vi "start.search.vi"(8 "error in (no error)":errorcluster, 9 "search dirs":path[](array[path]), 11 "comic_crawler in":refnum<class "comic_crawler.lvclass">) -> (0 "error out":errorcluster, 3 "comic_crawler out":refnum<class "comic_crawler.lvclass">)   [LabVIEW 2024, in "comic_crawler.lvclass"]
uses:
  comic_crawler.lvclass
  daemon.states--enum.ctl
  WebScraper/comic_class/comic_class.lvclass
  comic_crawler.lvclass/comic_crawler.ctl
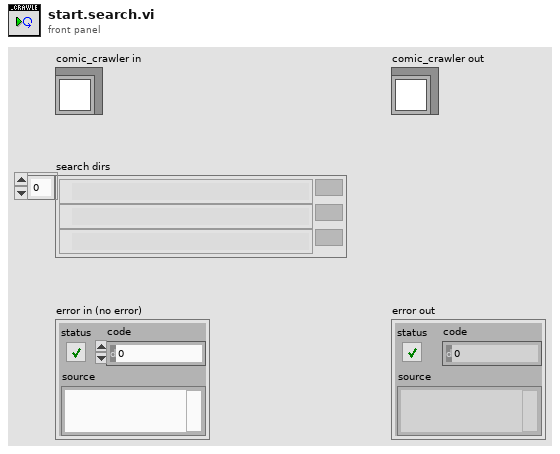
[diagram p1: front panel]
types:
  T1 = typedef "comic_crawler.lvclass/daemon.states--enum.ctl" = enum16{"start search", "idle", "set timer", "running", "stop search", "wait", "set delay", "shut down"}
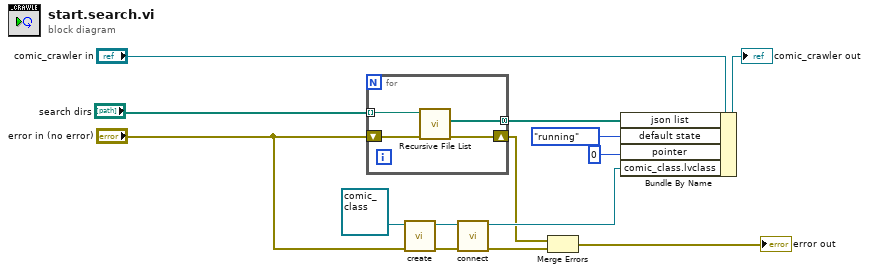
[diagram p0: block diagram]
diagram:
  n1 = for {
    tunnel: "search dirs" -> [w18] mode=indexing
    tunnel: [w17] -> w11 mode=concatenating
    shift-right: [w15] -> w3
    shift-left: "error in (no error)" -> [w16]
    n2 = call <vilib>:"Recursive File List.vi"("error in (no error)"=w16, "Folder Path"=w18) -> ("error out"=w15:errorcluster, "All Files in Dir"=w17:path[])  [unwired: 5 in, 3 out]
  }
  n3 = call "create.vi"("error in (no error)"="error in (no error)", "comic_class in"=refnum<class "comic_class.lvclass"> refnum ("comic_class.lvclass")) -> ("error out"=w8:errorcluster, "comic_class out"=w9:refnum<class "comic_class.lvclass">)  [unwired: 8 in]
  n4 = call-dynamic "connect.vi"("error in (no error)"=w8, "comic_class in"=w9) -> ("error out"=w4:errorcluster, "comic_class out"=w5:refnum<class "comic_class.lvclass">)  [unwired: 8 in]
  n5 = Merge Errors(w3, w4) -> (→"error out":errorcluster)
  n6 = Bundle By Name(cluster="comic_crawler in", "json list"=w11, "default state"=daemon.states--enum."running", "pointer"=0, "comic_class.lvclass"=w5) -> (→"comic_crawler out":refnum<class "comic_crawler.lvclass">)
